vi "Modify Config Templates.vi"() -> ()   [LabVIEW 2021]
uses:
  <vilib>/Utility/sysdir.llb/System Directory Type.ctl
panel:
  out "String":string
  out "error out":errorcluster
  out "text":string
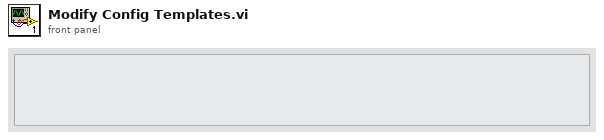
[diagram p1: front panel]
types:
  T1 = typedef "System Directory Type.ctl" = i32
  T2 = enum32{"invalid app kind", "Development System", "Run Time System", "Student Edition", "Embedded LabVIEW", "Evaluation", "Custom"}
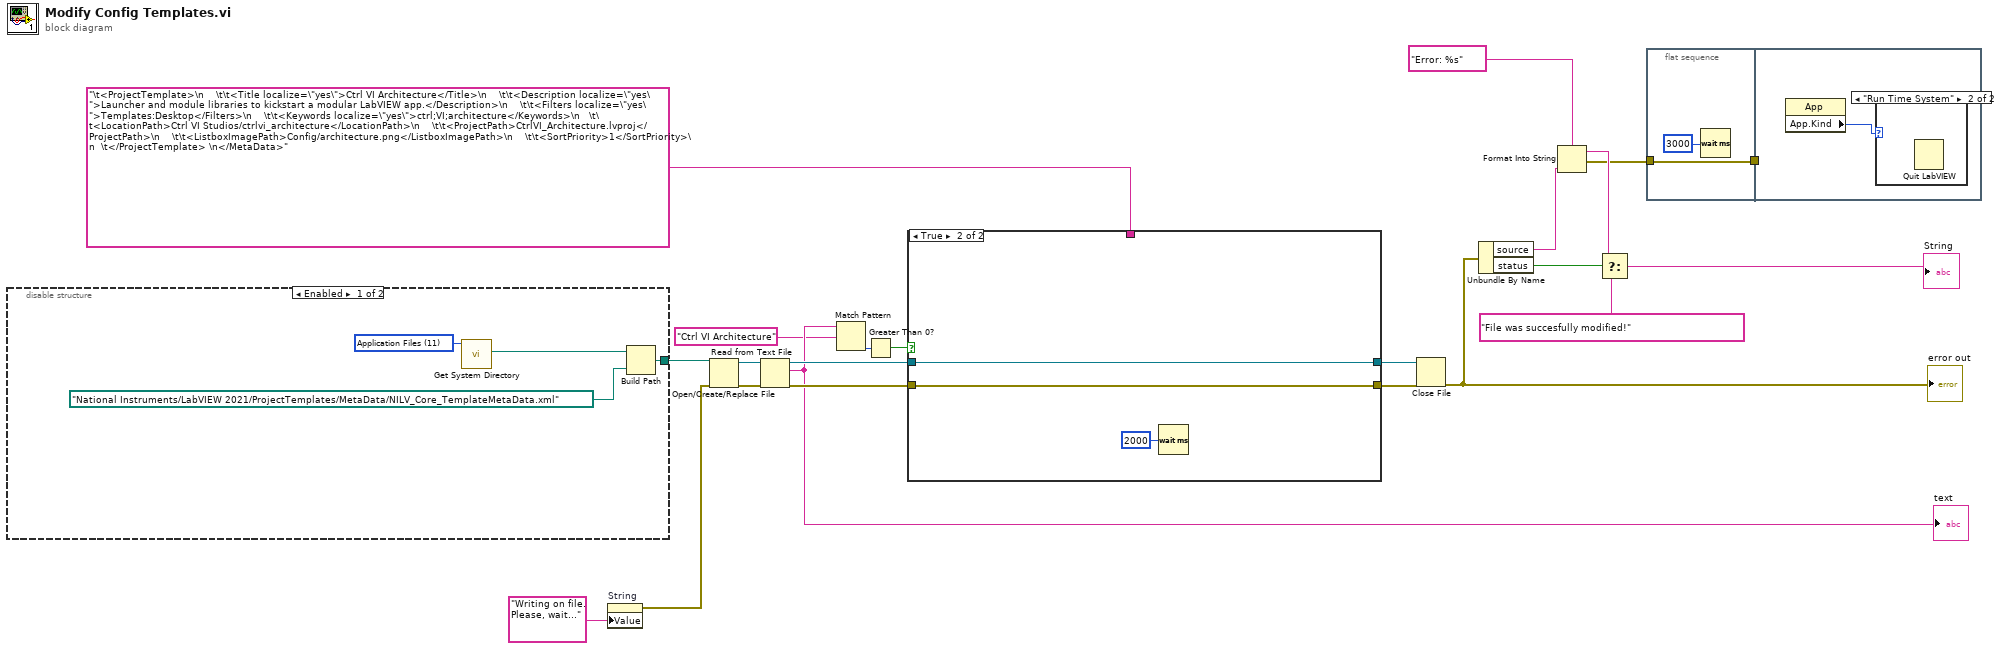
[diagram p0: block diagram]
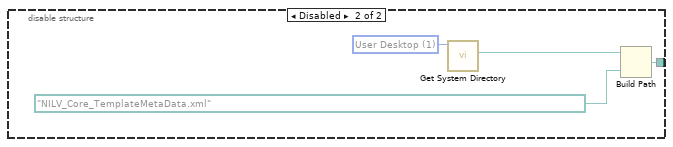
[diagram p3: hidden frame]
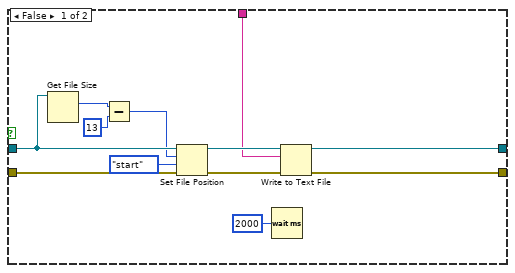
[diagram p4: hidden frame]
diagram:
  n1 = disable-structure shown="Enabled" {
    disable-tunnel: [w24 w28] -> w23
    frame Enabled {
      w27 = T1 11 items=["User Home"=0, "User Desktop"=1, "User Documents"=2, "User Application Data"=3, "User Preferences"=4, "User Temporary"=5, "Public Documents"=6, "Public Application Data"=7, "Public Preferences"=8, "Public Cache"=13, "System Core Libraries"=9, "System Installed Libraries"=10, "Application Files"=11, "Boot Volume Root"=12] ("system directory type")
      n2 = call <vilib>:"Get System Directory.vi"("system directory type"=w27) -> ("system directory"=w26:path)  [unwired: 10 in]
      n3 = Build Path(base path=w26, name or relative path=path "National Instruments/LabVIEW 2021/ProjectTemplates/MetaData/NILV_Core_TemplateMetaData.xml") -> (appended path=w24:path)
    }
    frame Disabled {
      w31 = T1 1 items=["User Home"=0, "User Desktop"=1, "User Documents"=2, "User Application Data"=3, "User Preferences"=4, "User Temporary"=5, "Public Documents"=6, "Public Application Data"=7, "Public Preferences"=8, "Public Cache"=13, "System Core Libraries"=9, "System Installed Libraries"=10, "Application Files"=11, "Boot Volume Root"=12] ("system directory type")
      n4 = call <vilib>:"Get System Directory.vi"("system directory type"=w31) -> ("system directory"=w30:path)  [unwired: 10 in]
      n5 = Build Path(base path=w30, name or relative path=path "NILV_Core_TemplateMetaData.xml") -> (appended path=w28:path)
    }
  }
  n6 = property on="String" class="Str"("Value"="Writing on file. Please, wait..." ("String")) -> (error out=w5:errorcluster)  [unwired: 2 in, 1 out]
  n7 = Open/Create/Replace File(file path (use dialog)=w23, error in=w5) -> (refnum out=w22:refnum<file>, error out=w21:errorcluster)  [unwired: 4 in, 1 out]
  n8 = Read from Text File(file (use dialog)=w22, error in=w21) -> (refnum out=w19:refnum<file>, text=w16:string, error out=w20:errorcluster)  [unwired: 2 in, 1 out]
  "text" <- w16
  n9 = Match Pattern(string=w16, regular expression="Ctrl VI Architecture") -> (offset past match=w14:i32)  [unwired: 1 in, 3 out]
  n10 = Greater Than 0?(x=w14) -> (x > 0?=w13:bool)
  n11 = case shown="True" w13 {
    tunnel: w20 -> [w43 w46]
    tunnel: w19 -> [w36 w45]
    tunnel: [w40 w46] -> w18
    tunnel: [w38 w45] -> w17
    tunnel: "\t<ProjectTemplate>\n    \t\t<Title localize=\"yes\">Ctrl VI Architecture</Title>\n    \t\t<Description localize=\"yes\">Launcher and module libraries to kickstart a modular LabVIEW app.</Description>\n    \t\t<Filters localize=\"yes\">Templates:Desktop</Filters>\n    \t\t<Keywords localize=\"yes\">ctrl;VI;architecture</Keywords>\n   \t\t<LocationPath>Ctrl VI Studios/ctrlvi_architecture</LocationPath>\n    \t\t<ProjectPath>CtrlVI_Architecture.lvproj</ProjectPath>\n    \t\t<ListboxImagePath>Config/architecture.png</ListboxImagePath>\n    \t\t<SortPriority>1</SortPriority>\n  \t</ProjectTemplate> \n</MetaData>" ("text") -> [w37 _]
    frame False {
      n12 = Get File Size(file=w36) -> (size (in bytes)=w35:i64)  [unwired: 1 in, 2 out]
      n13 = Subtract(x=w35, y=i64 13 ("offset (in bytes) (0)")) -> (x-y=w33:i64)
      n14 = Set File Position(offset (in bytes) (0)=w33, refnum=w36, from (0:start)=enum16{"start", "end", "current"}."start", error in=w43) -> (refnum out=w39:refnum<file>, error out=w42:errorcluster)
      n15 = Wait (ms)(milliseconds to wait=u32 2000) -> ()  [unwired: 1 out]
      n16 = Write to Text File(file (use dialog)=w39, text=w37, error in=w42) -> (refnum out=w38:refnum<file>, error out=w40:errorcluster)  [unwired: 1 in, 1 out]
    }
    frame True {
      n17 = Wait (ms)(milliseconds to wait=u32 2000) -> ()  [unwired: 1 out]
    }
  }
  n18 = Close File(refnum=w17, error in=w18) -> (error out=w3:errorcluster)  [unwired: 1 out]
  "error out" <- w3
  n19 = Unbundle By Name(w3) -> ("source"=w9:string, "status"=w11:bool)
  n20 = Format Into String(format string="Error: %s" ("String"), w9) -> (resulting string=w8:string, error out=w2:errorcluster)  [unwired: 2 in]
  n21 = Select(t=w8, s=w11, f="File was succesfully modified!" ("String")) -> (s? t:f=→"String":string)
  n22 = flat-sequence {
    tunnel: w2 -> [w47]
    tunnel: [w47] -> w1
    tunnel: w1 -> [_]
    frame #0 {
      n23 = Wait (ms)(milliseconds to wait=u32 3000) -> ()  [unwired: 1 out]
    }
    frame #1 {
      n24 = property class="App"() -> ("App.Kind"=w49:T2)  [unwired: 2 in, 2 out]
      n25 = case shown="\"Run Time System\"" w49 {
        frame "invalid app kind", Default {
        }
        frame "Run Time System" {
          n26 = Quit LabVIEW() -> ()  [unwired: 1 in]
        }
      }
    }
  }
